vi "DataTransmissionGlobals.vi"() -> ()   [LabVIEW 2009]
panel:
  in  "Stepwise Flag":bool
  in  "Channel Names":string[](array[string])
  in  "Port Number":dbl
  in  "Transmission State":T1(ring)
  in  "Notification Name":string="DataAvailableForTransmission"
  in  "Enabled":bool
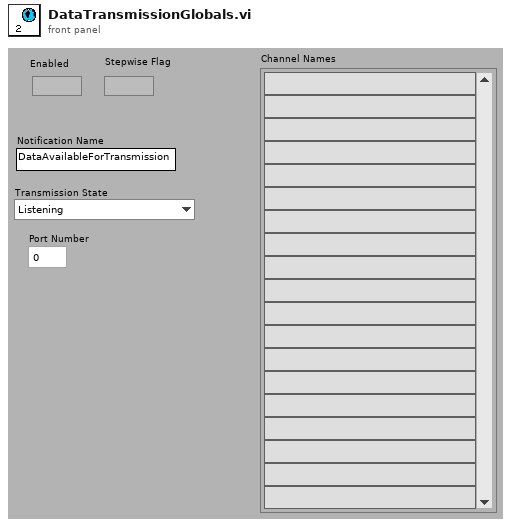
[diagram p1: front panel]
types:
  T1 = enum16{"Listening", "Initializing", "Transmitting", "Disconnecting"}
diagram:
